vi "Initialize.vi"(7 "Process ID":string, 8 "error in (no error)":errorcluster, 11 "FRTS Process in":refnum<class "FRTS Process.lvclass">) -> (0 "error out":errorcluster, 3 "FRTS Process out":refnum<class "FRTS Process.lvclass">)   [LabVIEW 2019, in "TimingDRV Engine.lvlib" / "FRTS Process.lvclass"]
uses:
  FRTS Process.lvclass
  C:/Users/XEnderMD/Desktop/CD Project Tools/Source/Engine/Parent Classes/Process/Process.lvclass
  Parent Classes/Process/Process.lvclass/Process.ctl
  FRTS Process.lvclass/FRTS Process.ctl
  <vilib>/NI VeriStand/Custom Device API/Get Item Property (I32).vi
  Parent Classes/TimerDRV Class/Methods/Configure TimerDRV Instances/Configure FreeRunning TimerDRV.vi
  Parent Classes/Process/Process.lvclass
  Parent Classes/TimerDRV Class/TimerDRV.lvclass
  <vilib>/NI VeriStand/Custom Device API/Custom Device API.lvlib
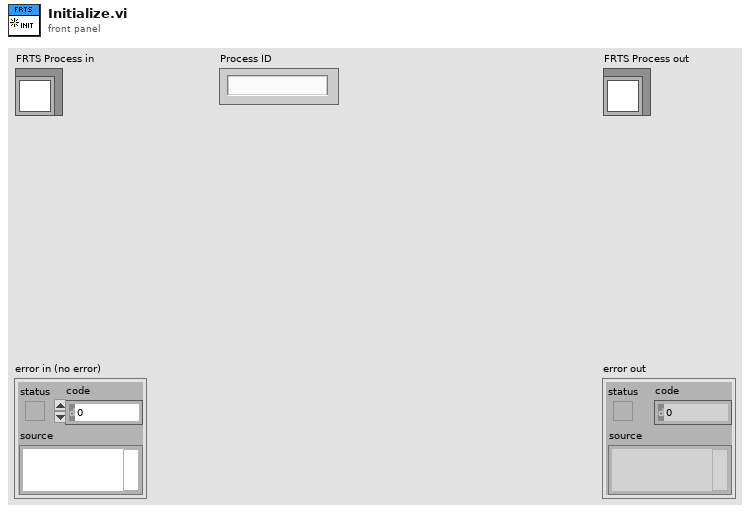
[diagram p1: front panel]
types:
  T1 = typedef "TimingDRV Engine.lvlib/Process.lvclass/Async Paramters.ctl" = cluster{"Device Reference":T2, "Device Clock":string, "Device Inputs FIFO":refnum<k33>, "Device Outputs FIFO":refnum<k33>, "CD Engine Event Ref":T3}
  T2 = typedef "Custom Device API.lvlib/Custom Device Item Ref.ctl" = u64
  T3 = typedef "Custom Device API.lvlib/Custom Device Engine Event Ref.ctl" = refnum<event-registration>
  T4 = typedef "Custom Device API.lvlib/Custom Device Target Type.ctl" = enum16{"PharLap", "VxWorks", "Windows", "Linux_32_ARM", "Linux_x64"}
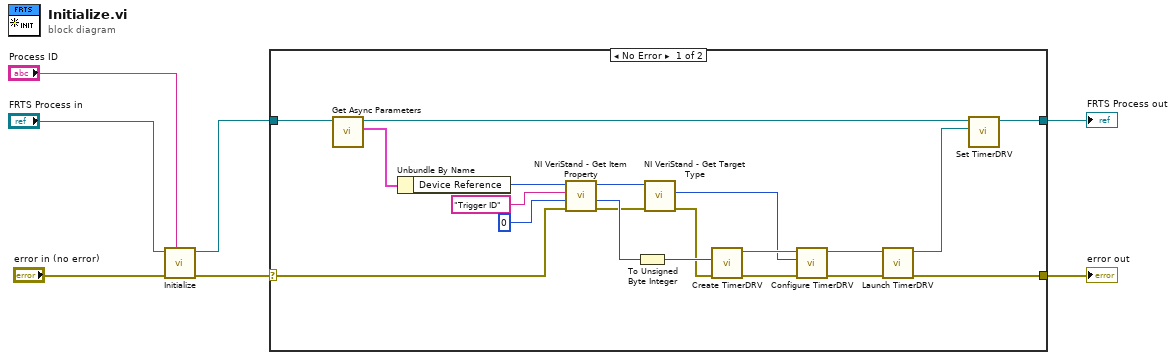
[diagram p0: block diagram]
diagram:
  n1 = call-parent "Initialize.vi"("Process ID"="Process ID", "error in (no error)"="error in (no error)", "Process in"="FRTS Process in") -> ("error out"=w4:errorcluster, "Process out"=w3:refnum<class "FRTS Process.lvclass">)  [unwired: 7 in]
  n2 = case shown="No Error" w4 {
    selector: w4 -> [w15 w28]
    tunnel: w3 -> [w27 w29]
    tunnel: [w9 w29] -> w1
    tunnel: [w11 w28] -> w2
    frame No Error {
      n3 = call "Get Async Parameters.vi"("Process in"=w27) -> ("Async Parameters"=w26:T1, "Process out"=w10:refnum<class "FRTS Process.lvclass">)  [unwired: 9 in]
      n4 = Unbundle By Name(w26) -> ("Device Reference"=w25:T2)
      n5 = call-poly <vilib>:"NI VeriStand - Get Item Property.vi"("error in (no error)"=w15, "Default Value"=0, "Property Name"="Trigger ID", "Item Ref in"=w25) -> ("error out"=w16:errorcluster, "Value"=w22:i32, "Item Ref out"=w18:T2)  [unwired: 4 in, 1 out]
      n6 = To Unsigned Byte Integer(number=w22) -> (unsigned 8bit integer=w21:u8)
      n7 = call <vilib>:"NI VeriStand - Get Target Type.vi"("error in (no error)"=w16, "Item Ref in"=w18) -> ("error out"=w14:errorcluster, "Target Type"=w17:T4)  [unwired: 7 in, 1 out]
      n8 = call "Create TimerDRV.vi"("error in (no error)"=w14, "Trigger ID"=w21) -> ("error out"=w20:errorcluster, "TimerDRV out"=w19:refnum<class "TimerDRV.lvclass">)  [unwired: 8 in]
      n9 = call-poly "Configure TimerDRV.vi"("error in (no error)"=w20, "Target Type"=w17, "TimerDRV in"=w19) -> ("error out"=w13:errorcluster, "TimerDRV out"=w12:refnum<class "TimerDRV.lvclass">)  [unwired: 7 in]
      n10 = call "Launch TimerDRV.vi"("error in (no error)"=w13, "TimerDRV in"=w12) -> ("error out"=w11:errorcluster, "TimerDRV out"=w8:refnum<class "TimerDRV.lvclass">)  [unwired: 8 in]
      n11 = call "Set TimerDRV.vi"("TimingDRV Engine.lvlib:TimerDRV.lvclass"=w8, "FRTS Process in"=w10) -> ("FRTS Process out"=w9:refnum<class "FRTS Process.lvclass">)  [unwired: 9 in]
    }
    frame Error {
    }
  }
  "error out" <- w2
  "FRTS Process out" <- w1
